vi "Get XML Attribute.vi"(8 "error in":errorcluster, 10 "Attribute Name":string, 11 "XML Node":refnum<k20>) -> (0 "error out":errorcluster, 2 "Attribute Value":string, 3 "XML Node out":refnum<k20>)   [LabVIEW 2024, in "Parser.lvlib"]
uses:
  Parser.lvlib
  <vilib>/xml/Close Reference(Node).vi
  <vilib>/xml/Close Reference(NNMap).vi
  <resource>/objmgr/DOMUserDefRef.rc
  <vilib>/xml/NI_XML.lvlib
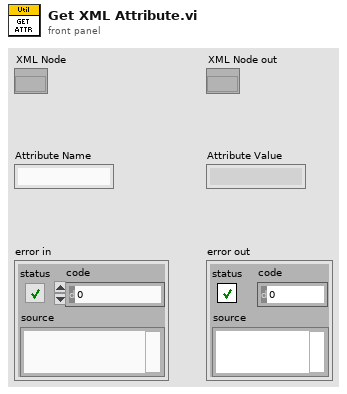
[diagram p1: front panel]
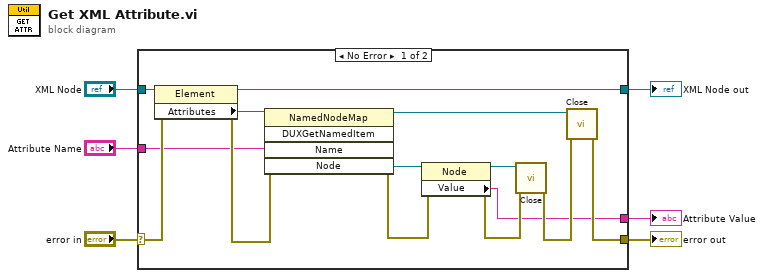
[diagram p0: block diagram]
diagram:
  n1 = case shown="No Error" "error in" {
    selector: "error in" -> [w17 w22]
    tunnel: [w15 w22] -> w6
    tunnel: "XML Node" -> [w14 w21]
    tunnel: "Attribute Name" -> [w12 _]
    tunnel: [w10 _] -> w2
    tunnel: [w8 w21] -> w1
    frame No Error {
      n2 = property on="Property Node" class="Element"(reference=w14, error in=w17) -> (reference out=w8:refnum<k20>, error out=w20:errorcluster, "Attributes"=w13:refnum<k20>)
      n3 = invoke on="Invoke Node" class="NamedNodeMap" method="DUXGetNamedItem"(reference=w13, error in=w20, "Name"=w12) -> (reference out=w7:refnum<k20>, error out=w19:errorcluster, "Node"=w11:refnum<k20>)  [unwired: 2 in, 2 out]
      n4 = property on="Property Node" class="Node"(reference=w11, error in=w19) -> (reference out=w9:refnum<k20>, error out=w18:errorcluster, "Value"=w10:string)
      n5 = call-poly <vilib>:"Close.vi"("error in (no error)"=w18, "node"=w9) -> ("error out"=w16:errorcluster)  [unwired: 7 in]
      n6 = call-poly <vilib>:"Close.vi"("error in (no error)"=w16, "named node map"=w7) -> ("error out"=w15:errorcluster)  [unwired: 7 in]
    }
    frame Error {
    }
  }
  "Attribute Value" <- w2
  "XML Node out" <- w1
  "error out" <- w6
